vi "Measure5314x.vi"() -> ()   [LabVIEW 2011]
panel:
  in  "Measurement (0: Frequency 1)":T1(ring)=enum."Frequency 2"
  out "error out":errorcluster
  out "return count":u32
  out "Readings":string[](array[string])
  in  "Number of Readings":dbl=5.0 min=2.0 max=10.0 step=2.0
  in  "VISA resource name":refnum<visa-resource-name>
  in  "ID Query":bool
  in  "error in (no error)":errorcluster
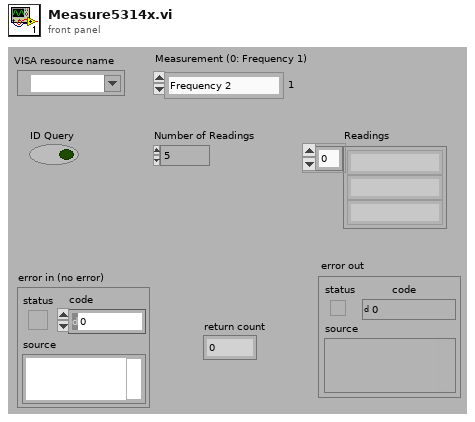
[diagram p1: front panel]
types:
  T1 = enum16{"Frequency 1", "Frequency 2", "Power", "Voltage"}
  T2 = cluster{"status":bool, "code":i32, "VI Name":string}
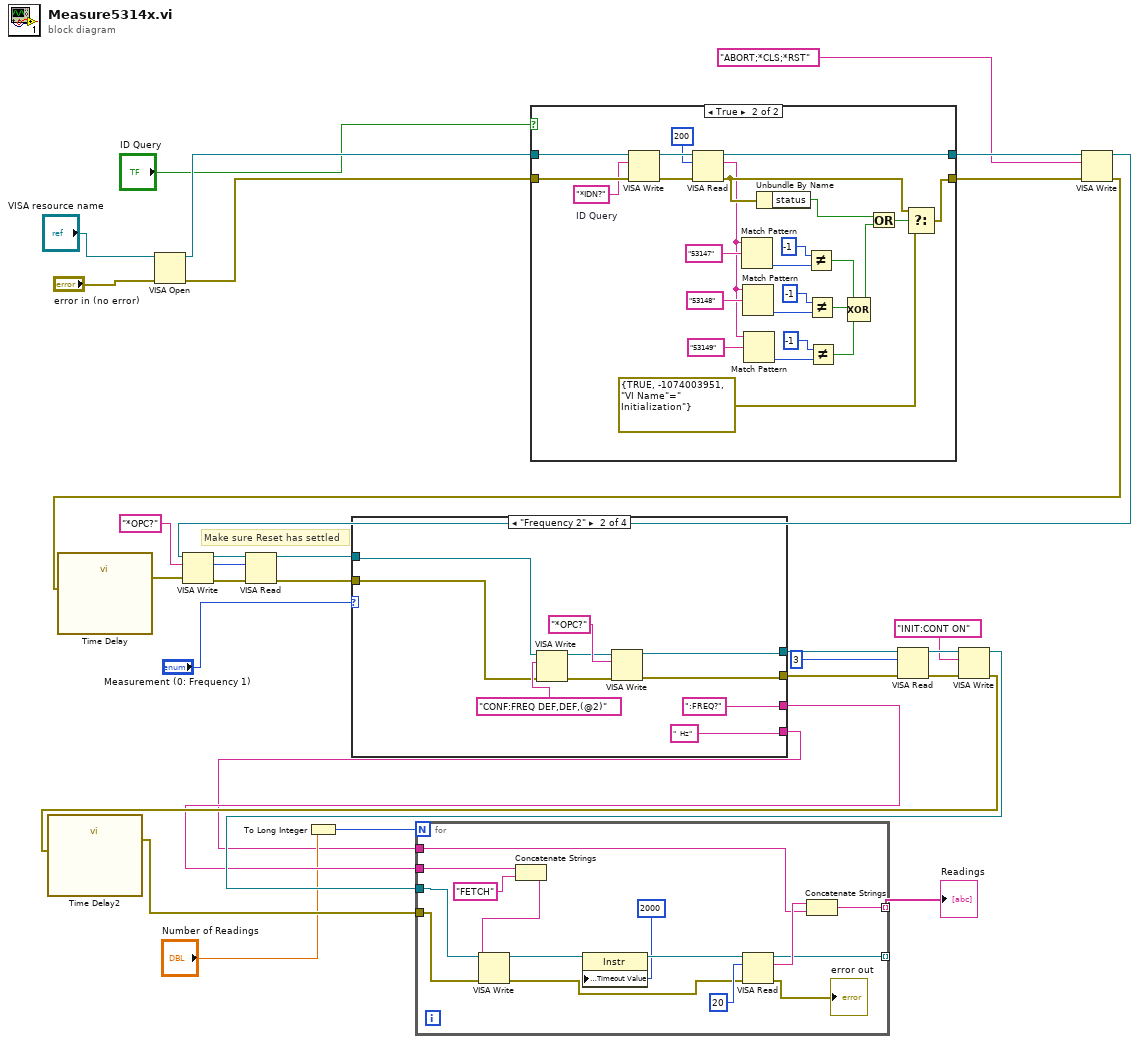
[diagram p0: block diagram]
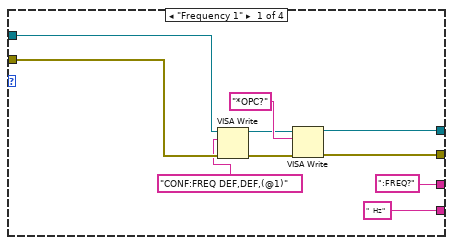
[diagram p2: hidden frame]
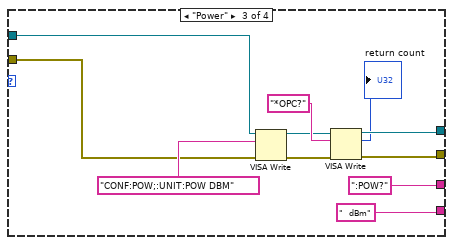
[diagram p3: hidden frame]
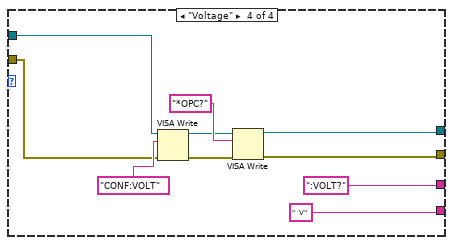
[diagram p4: hidden frame]
diagram:
  # "Make sure Reset has settled"
  n1 = VISA Open(error in (no error)="error in (no error)", VISA resource name="VISA resource name") -> (VISA resource name=w32:refnum<visa-resource-name>, error out=w28:errorcluster)  [unwired: 3 out]
  n2 = To Long Integer(number="Number of Readings") -> (32bit integer=w2:i32)
  n3 = case shown="True" "ID Query" {
    tunnel: [w33 w60] -> w26
    tunnel: [w34 w59] -> w27
    tunnel: w32 -> [w34 w49]
    tunnel: w28 -> [w33 w50]
    frame False {
    }
    frame True {
      w48 = "*IDN?"  # ID Query
      n4 = VISA Write(VISA resource name=w49, write buffer=w48, error in (no error)=w50) -> (VISA resource name out=w51:refnum<visa-resource-name>, error out=w53:errorcluster)  [unwired: 1 out]
      n5 = VISA Read(VISA resource name=w51, byte count=u32 200, error in (no error)=w53) -> (VISA resource name out=w59:refnum<visa-resource-name>, read buffer=w35:string, error out=w52:errorcluster)  [unwired: 1 out]
      n6 = Match Pattern(string=w35, regular expression="53147") -> (offset past match=w58:i32)  [unwired: 4 out]
      n7 = Match Pattern(string=w35, regular expression="53148") -> (offset past match=w45:i32)  [unwired: 4 out]
      n8 = Match Pattern(string=w35, regular expression="53149") -> (offset past match=w42:i32)  [unwired: 4 out]
      n9 = Unbundle By Name(w52) -> ("status"=w55:bool)
      n10 = Not Equal?(x=-1, y=w58) -> (x != y?=w39:bool)
      n11 = Not Equal?(x=-1, y=w45) -> (x != y?=w38:bool)
      n12 = Not Equal?(x=-1, y=w42) -> (x != y?=w37:bool)
      n13 = Compound Arithmetic op=XOR(w39, w38, w37) -> (w36:bool)
      n14 = Or(x=w55, y=w36) -> (x .or. y?=w54:bool)
      n15 = Select(t=w52, s=w54, f=cluster{bool, i32, "VI Name":string} {TRUE, -1074003951, "VI Name"=" Initialization"}) -> (s? t:f=w60:T2)
    }
  }
  n16 = VISA Write(VISA resource name=w27, write buffer="ABORT;*CLS;*RST", error in (no error)=w26) -> (VISA resource name out=w21:refnum<visa-resource-name>, error out=w24:errorcluster)  [unwired: 1 out]
  n17 = call "Time Delay"("error in (no error)"=w24) -> ("error out"=w22:errorcluster)  [unwired: 1 in, 9 out]
  n18 = VISA Write(VISA resource name=w21, write buffer="*OPC?", error in (no error)=w22) -> (VISA resource name out=w18:refnum<visa-resource-name>, return count=w19:u32, error out=w20:errorcluster)
  n19 = VISA Read(VISA resource name=w18, byte count=w19, error in (no error)=w20) -> (VISA resource name out=w16:refnum<visa-resource-name>, error out=w17:errorcluster)  [unwired: 2 out]
  n20 = case shown="\"Frequency 2\"" "Measurement (0: Frequency 1)" {
    tunnel: w17 -> [w69 w75 w86 w92]
    tunnel: w16 -> [w70 w76 w87 w93]
    tunnel: [w64 w74 w85 w95] -> w12
    tunnel: [w63 w73 w84 w94] -> w11
    tunnel: [":FREQ?" ":FREQ?" ":POW?" ":VOLT?"] -> w6
    tunnel: ["  Hz" "  Hz" "  dBm" "  V"] -> w1
    frame "Frequency 1" {
      n21 = VISA Write(VISA resource name=w70, write buffer="CONF:FREQ DEF,DEF,(@1)", error in (no error)=w69) -> (VISA resource name out=w66:refnum<visa-resource-name>, error out=w65:errorcluster)  [unwired: 1 out]
      n22 = VISA Write(VISA resource name=w66, write buffer="*OPC?", error in (no error)=w65) -> (VISA resource name out=w64:refnum<visa-resource-name>, error out=w63:errorcluster)  [unwired: 1 out]
    }
    frame "Frequency 2" {
      n23 = VISA Write(VISA resource name=w76, write buffer="CONF:FREQ DEF,DEF,(@2)", error in (no error)=w75) -> (VISA resource name out=w78:refnum<visa-resource-name>, error out=w77:errorcluster)  [unwired: 1 out]
      n24 = VISA Write(VISA resource name=w78, write buffer="*OPC?", error in (no error)=w77) -> (VISA resource name out=w74:refnum<visa-resource-name>, error out=w73:errorcluster)  [unwired: 1 out]
    }
    frame "Power" {
      n25 = VISA Write(VISA resource name=w87, write buffer="CONF:POW;:UNIT:POW DBM", error in (no error)=w86) -> (VISA resource name out=w89:refnum<visa-resource-name>, error out=w88:errorcluster)  [unwired: 1 out]
      n26 = VISA Write(VISA resource name=w89, write buffer="*OPC?", error in (no error)=w88) -> (VISA resource name out=w85:refnum<visa-resource-name>, return count=→"return count":u32, error out=w84:errorcluster)
    }
    frame "Voltage" {
      n27 = VISA Write(VISA resource name=w93, write buffer="CONF:VOLT", error in (no error)=w92) -> (VISA resource name out=w99:refnum<visa-resource-name>, error out=w98:errorcluster)  [unwired: 1 out]
      n28 = VISA Write(VISA resource name=w99, write buffer="*OPC?", error in (no error)=w98) -> (VISA resource name out=w95:refnum<visa-resource-name>, error out=w94:errorcluster)  [unwired: 1 out]
    }
  }
  n29 = VISA Read(VISA resource name=w12, byte count=u32 3, error in (no error)=w11) -> (VISA resource name out=w14:refnum<visa-resource-name>, error out=w15:errorcluster)  [unwired: 2 out]
  n30 = VISA Write(VISA resource name=w14, write buffer="INIT:CONT ON", error in (no error)=w15) -> (VISA resource name out=w8:refnum<visa-resource-name>, error out=w10:errorcluster)  [unwired: 1 out]
  n31 = call "Time Delay2"("error in (no error)"=w10) -> ("error out"=w7:errorcluster)  [unwired: 1 in, 9 out]
  n32 = for {
    N: w2 -> [_]
    tunnel: w8 -> [w115]
    tunnel: w7 -> [w116]
    tunnel: w1 -> [w109]
    tunnel: w6 -> [w113]
    tunnel: [w108] -> w5 mode=indexing
    tunnel: [w107] -> _ mode=indexing
    n33 = Concatenate Strings(w113, "FETCH" ("string")) -> (w112:string)
    n34 = VISA Write(VISA resource name=w115, write buffer=w112, error in (no error)=w116) -> (VISA resource name out=w105:refnum<visa-resource-name>, error out=w102:errorcluster)  [unwired: 1 out]
    n35 = property class="Instr"(reference=w105, "General Settings:Timeout Value"=u32 2000) -> (reference out=w104:refnum<visa-resource-name>)  [unwired: 1 in, 1 out]
    n36 = VISA Read(VISA resource name=w104, byte count=u32 20, error in (no error)=w102) -> (VISA resource name out=w107:refnum<visa-resource-name>, read buffer=w110:string, error out=→"error out":errorcluster)  [unwired: 1 out]
    n37 = Concatenate Strings(w110, w109) -> (w108:string)
  }
  "Readings" <- w5
